vi "Write Account.vi"(8 "error in (no error)":errorcluster, 10 "Account":string, 11 "AReceipt in":refnum<class "AReceipt.lvclass">) -> (0 "error out":errorcluster, 3 "AReceipt out":refnum<class "AReceipt.lvclass">)   [LabVIEW 2020, in "AReceipt.lvclass"]
uses:
  AReceipt.lvclass
  AReceipt.lvclass/AReceipt.ctl
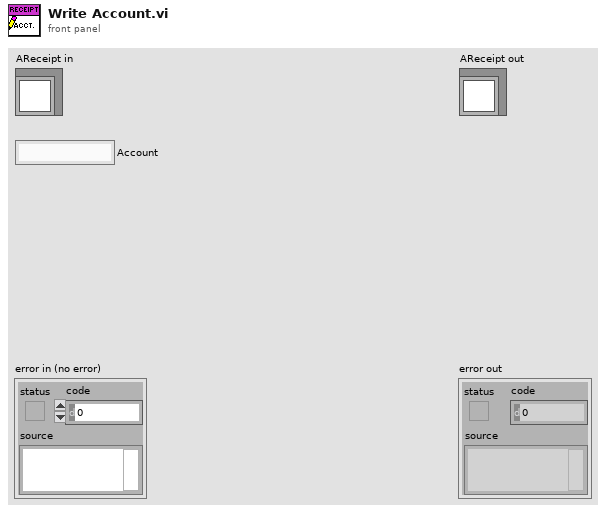
[diagram p1: front panel]
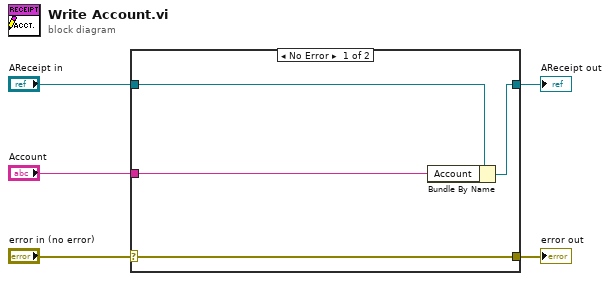
[diagram p0: block diagram]
diagram:
  n1 = case shown="No Error" "error in (no error)" {
    selector: "error in (no error)" -> [w9 w10]
    tunnel: [w9 w10] -> w4
    tunnel: [w7 w11] -> w2
    tunnel: "AReceipt in" -> [w8 w11]
    tunnel: "Account" -> [w6 _]
    frame No Error {
      n2 = Bundle By Name(cluster=w8, "Account"=w6) -> (w7:refnum<class "AReceipt.lvclass">)
    }
    frame Error {
    }
  }
  "error out" <- w4
  "AReceipt out" <- w2
